vi "task333.vi"() -> ()   [LabVIEW 2024]
uses:
  4e3d31d6-c078-42b0-8f13-7a43813e1c35.vi
  89b9b800-7582-48e6-9300-e7a78ae21f87.vi
panel:
  in  "noise amp":dbl
  in  "signal frequency":dbl
  in  "sampling frequency":dbl
  out "Iteration number":i32
  out "out":dbl
  out "4":dbl
  out "2":dbl
  out "3":dbl
  out "1":dbl
  out "0":dbl
  in  "Wait time":dbl=1.0
  in  "stop":bool
  out "Random Numbers":cluster{dbl, dbl}(graph)
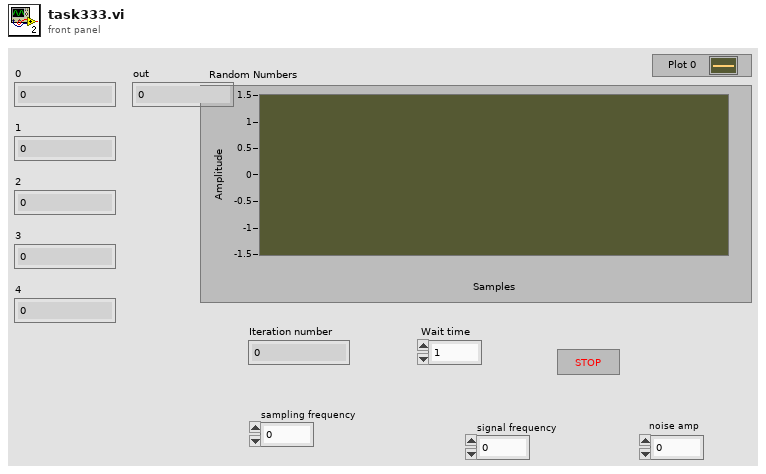
[diagram p1: front panel]
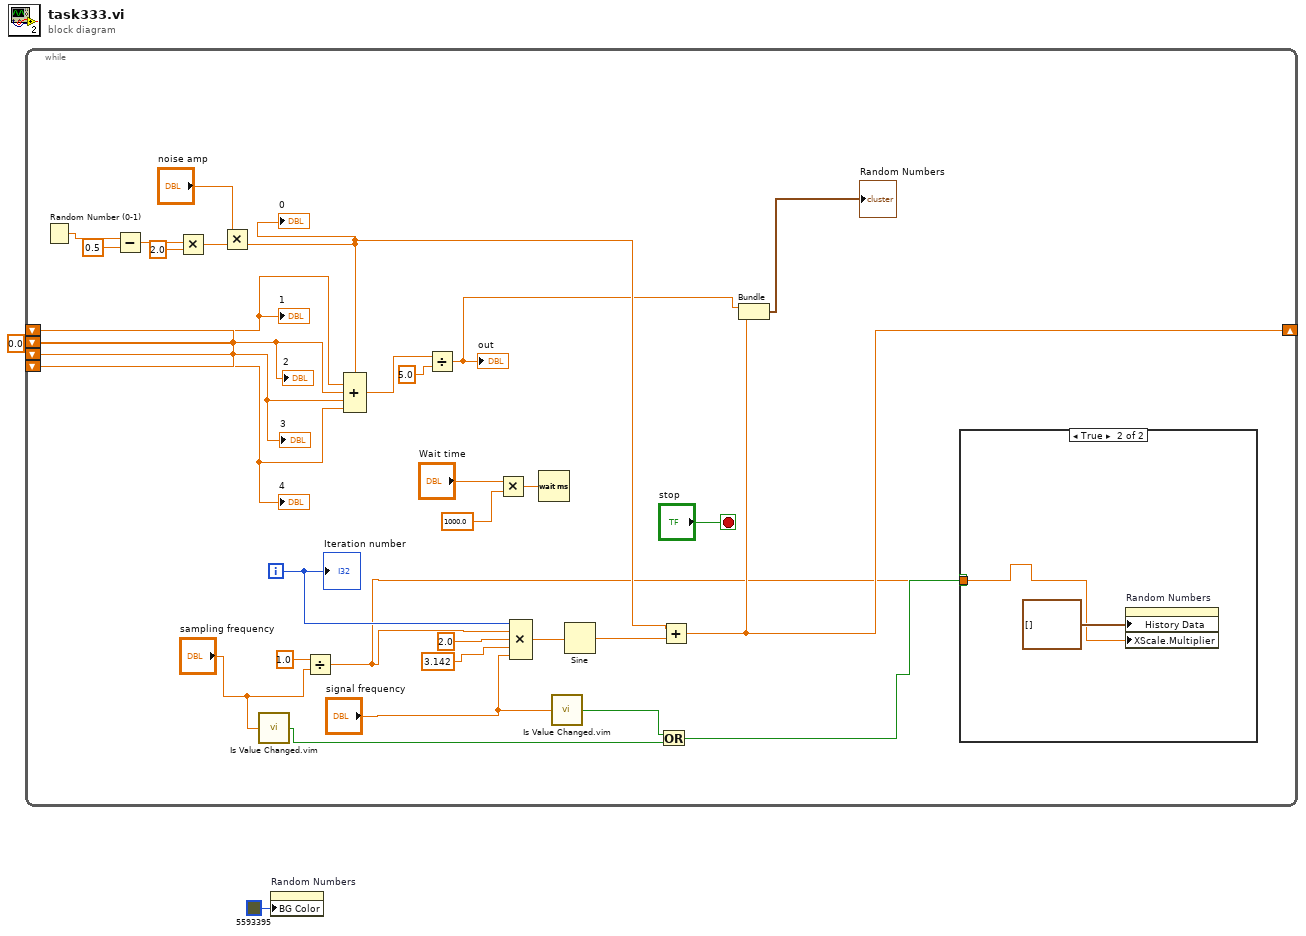
[diagram p0: block diagram]
diagram:
  w2 = 0.0 ("number: 0 to 1")
  n1 = while {
    shift-right: [w11] -> _
    shift-left: w2 -> [w29]
    shift-left: w2 -> [w28]
    shift-left: w2 -> [w27]
    shift-left: w2 -> [w26]
    i -> [w25]
    stop <- "stop" stop-if-true
    n2 = Random Number (0-1)() -> (number: 0 to 1=w20:dbl)
    n3 = Subtract(x=w20, y=0.5) -> (x-y=w18:dbl)
    n4 = Multiply(x=w18, y=2.0) -> (x*y=w16:dbl)
    n5 = Multiply(x="noise amp", y=w16) -> (x*y=w13:dbl)
    "0" <- w13
    n6 = call "Is Value Changed.vim"("value"="sampling frequency") -> ("changed or first call?"=w7:bool)
    n7 = Divide(x=1.0, y="sampling frequency") -> (x/y=w3:dbl)
    n8 = Compound Arithmetic op=ADD(w13, w29, w28, w27, w26) -> (w30:dbl)
    n9 = Divide(x=w30, y=5.0) -> (x/y=w12:dbl)
    "out" <- w12
    n10 = Multiply(x="Wait time", y=1000.0) -> (x*y=w4:dbl)
    n11 = Compound Arithmetic op=MULTIPLY(w25, w3, 2.0 ("value"), 3.142 ("value"), "signal frequency") -> (w21:dbl)
    n12 = Wait (ms)(milliseconds to wait=w4) -> ()  [unwired: 1 out]
    n13 = call "Is Value Changed.vim"("value"="signal frequency") -> ("changed or first call?"=w5:bool)
    n14 = Sine(x=w21) -> (sin(x)=w14:dbl)
    n15 = Or(x=w5, y=w7) -> (x .or. y?=w9:bool)
    n16 = Add(x=w13, y=w14) -> (x+y=w11:dbl)
    n17 = Bundle(w12, w11) -> (→"Random Numbers":cluster{dbl, dbl})  [unwired: 1 in]
    n18 = case shown="True" w9 {
      tunnel: w3 -> [_ w35]
      frame False {
      }
      frame True {
        n19 = property on="Random Numbers" class="WFChart (strict)"("History Data"=cluster{dbl, dbl}[] [], "XScale.Multiplier"=w35) -> ()  [unwired: 2 in, 2 out]
      }
    }
    "1" <- w29
    "3" <- w27
    "2" <- w28
    "4" <- w26
    "Iteration number" <- w25
  }
  n20 = property on="Random Numbers" class="WFChart (strict)"("BG Color"=u32 5593395 ("Plot Area:Colors:BG Color")) -> ()  [unwired: 2 in, 2 out]
